vi "Check B button.vi"(8 "error in (no error)":errorcluster, 11 "RDS Local Remote Actor in":refnum<class "RDS Local Remote Actor.lvclass">) -> (0 "error out":errorcluster, 3 "RDS Local Remote Actor out":refnum<class "RDS Local Remote Actor.lvclass">)   [LabVIEW 2015, in "RDS Local Remote Actor.lvlib" / "RDS Local Remote Actor.lvclass"]
uses:
  RDS Local Remote Actor.lvclass
  RDS Local Remote Actor.lvclass/RDS Local Remote Actor.ctl
  Libraries/RDS Child Messages/Controller Message/Controller Message Type.ctl
  Libraries/RDS Child Messages/Controller Message/Controller Message.lvclass
  RDS Parent Actor/RDS Parent Actor/RDS Parent Actor.lvclass
  RDS Controller Actor/RDS Controller Actor/RDS Controller Actor.lvlib
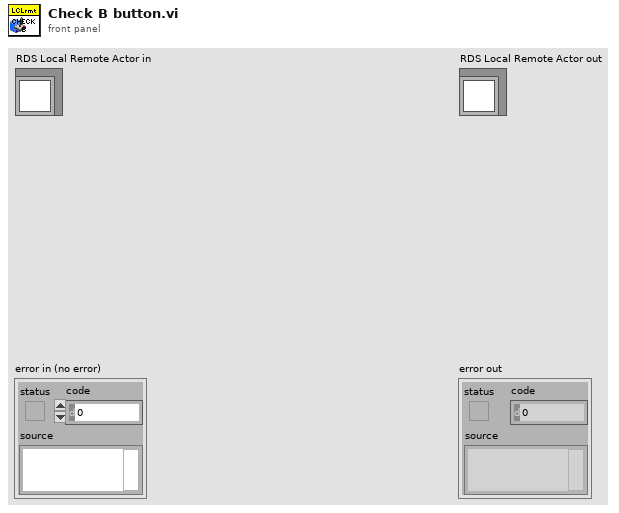
[diagram p1: front panel]
types:
  T1 = typedef "RDS Child Messages.lvlib/Controller Message.lvclass/Controller Message Type.ctl" = enum16{"Control Relinquish Request", "Control Relinquish Command", "Control Request", "Control Granted"}
  T2 = typedef "RDS Controller Actor.lvlib/Controller.ctl" = enum16{"Idle", "Local Remote Control", "Shore Remote Control", "Mission Control"}
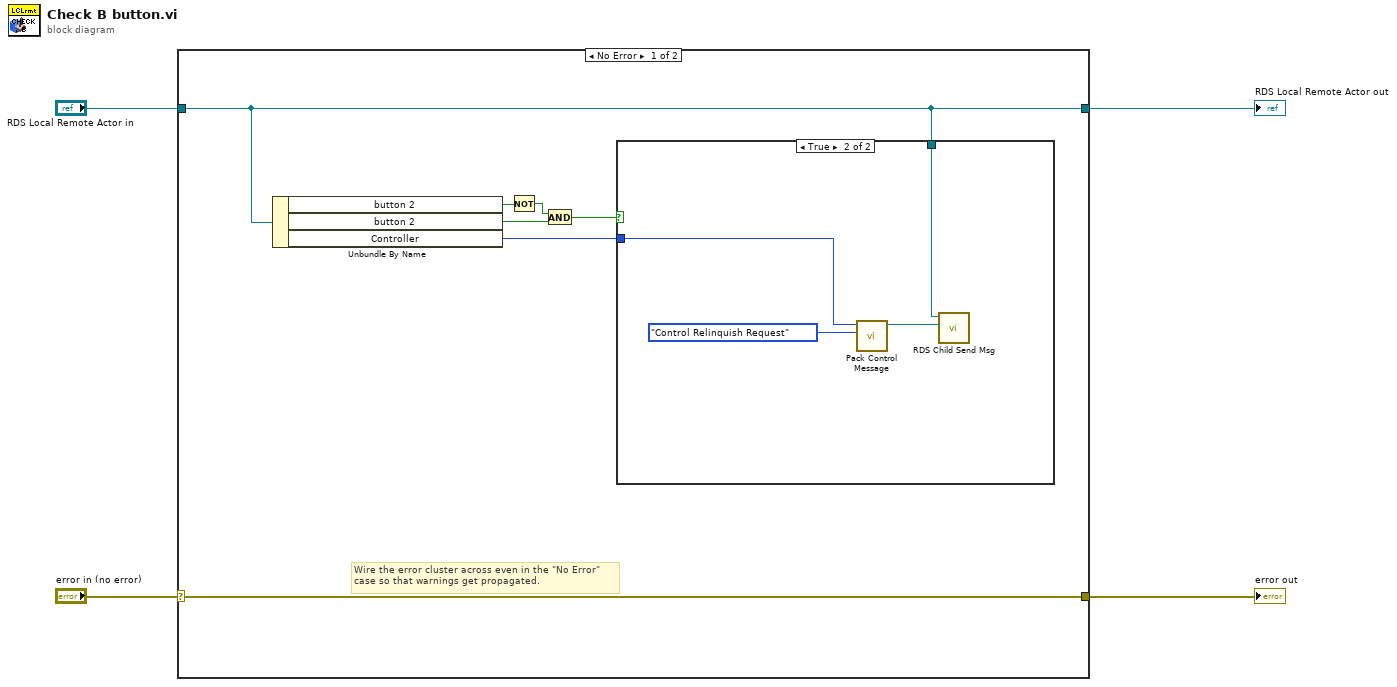
[diagram p0: block diagram]
diagram:
  n1 = case shown="No Error" "error in (no error)" {
    selector: "error in (no error)" -> [w11 w17]
    tunnel: [w11 w17] -> w3
    tunnel: [w6 w16] -> w1
    tunnel: "RDS Local Remote Actor in" -> [w6 w16]
    frame No Error {
      # "Wire the error cluster across even in the \"No Error\"\ncase so that warnings get propagated."
      n2 = Unbundle By Name(w6) -> ("button 2"=w10:bool, "button 2"=w8:bool, "Controller"=w5:T2)
      n3 = Not(x=w10) -> (.not. x?=w9:bool)
      n4 = And(x=w9, y=w8) -> (x .and. y?=w7:bool)
      n5 = case shown="True" w7 {
        tunnel: w6 -> [_ w14]
        tunnel: w5 -> [_ w13]
        frame False {
        }
        frame True {
          n6 = call "Pack Control Message.vi"("Controller Message Type"=Controller_Message_Type."Control Relinquish Request", "Controller"=w13) -> ("Controller Message out"=w15:refnum<class "Controller Message.lvclass">)  [unwired: 9 in]
          n7 = call "RDS Child Send Msg.vi"("RDS Message"=w15, "RDS Parent Actor in"=w14) -> ()  [unwired: 8 in, 2 out]
        }
      }
    }
    frame Error {
    }
  }
  "error out" <- w3
  "RDS Local Remote Actor out" <- w1
